vi "Create Database Item.vi"(8 "error in (no error)":errorcluster, 10 "type id":u32, 11 "eLab in":refnum<class "PL eLabFTW Client.lvclass">) -> (0 "error out":errorcluster, 2 "database item id":u32, 3 "eLab out":refnum<class "PL eLabFTW Client.lvclass">)   [LabVIEW 2015, in "PL eLabFTW Client.lvclass"]
doc: "Creates new database item of the specified type and returns new item id."
uses:
  PL eLabFTW Client.lvclass
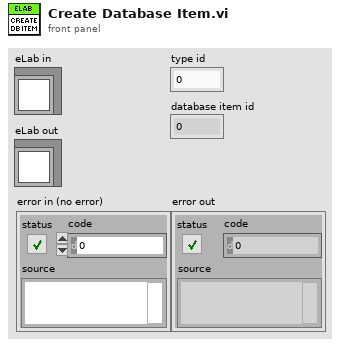
[diagram p1: front panel]
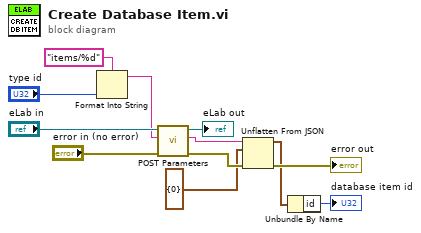
[diagram p0: block diagram]
diagram:
  n1 = Format Into String(format string="items/%d", "type id") -> (resulting string=w7:string)  [unwired: 2 in, 1 out]
  n2 = call "POST Parameters.vi"("error in (no error)"="error in (no error)", "relative URL"=w7, "eLab in"="eLab in") -> ("error out"=w6:errorcluster, "response body"=w2:string, "eLab out"=→"eLab out":refnum<class "PL eLabFTW Client.lvclass">)  [unwired: 6 in]
  n3 = Unflatten From JSON(JSON string=w2, type and defaults=cluster{"id":u32} {"id"=0}, error in (no error)=w6) -> (value=w3:cluster{"id":u32}, error out=→"error out":errorcluster)  [unwired: 4 in]
  n4 = Unbundle By Name(w3) -> ("id"=→"database item id":u32)
